vi "Actor Core.vi"(8 "error in":errorcluster, 11 "Linear Research in":refnum<class "Linear Research.lvclass">) -> (0 "error out":errorcluster, 3 "Actor out":refnum<class "Actor.lvclass">)   [LabVIEW 2015, in "Linear Research.lvclass"]
doc: "(<B>Filename</B>: Actor Framework.lvlib:Actor.lvclass:Actor Core.vi)\n\nReceives messages to the actor, reacts to them, and initiates any error handling that may shut the actor down.\n\nDescendant classes may override this VI to append parallel tasks for the actor to complete while it handles messages. Overrides use the Call Parent Method node."
uses:
  Linear Research.lvclass
  <vilib>/ActorFramework/Actor/Actor.lvclass
  Linear Research Parameters.ctl
  Meter/Meter.lvclass
panel:
  in  "Parameters":T1={"Scan  Channels"=[], "Merge scan with"="Temperature"}
  # "If list is empty - will not use scanner option"
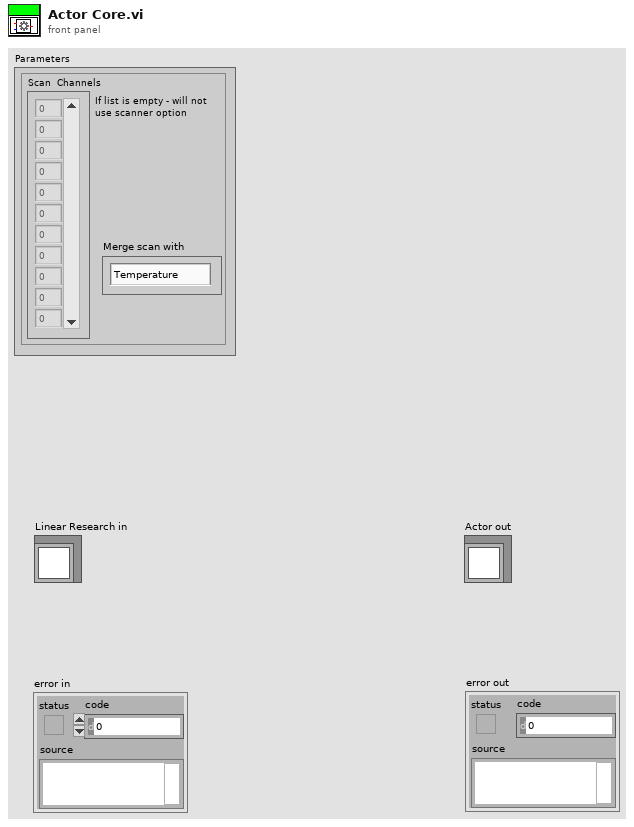
[diagram p1: front panel]
types:
  T1 = typedef "Linear Research Parameters.ctl" = cluster{"Scan  Channels":i32[], "Merge scan with":string}
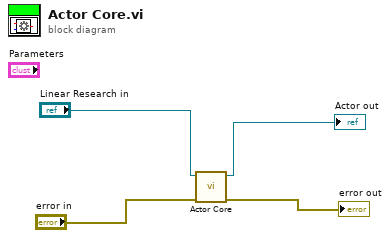
[diagram p0: block diagram]
diagram:
  n1 = call-parent "Actor Core.vi"("error in"="error in", "Meter in"="Linear Research in") -> ("error out"=→"error out":errorcluster, "Actor out"=→"Actor out":refnum<class "Actor.lvclass">)  [unwired: 8 in]
